vi "OAT Timebase Plot (Vector Data).vi"(0 "magnitudes":T3(array[cluster]) {"magnitude" format="%.2f"; "time/rev/rpm" format="%.2f"}, 2 "order to display":dbl=1.0 format="%.2f", 5 "phases [phase lag]":cluster{"time/rev/rpm":dbl[], "phase":dbl[]}[](array[cluster]) {"phase" format="%.2f"; "time/rev/rpm" format="%.2f"}, 7 "samples/rev wanted":i32=64, 9 "revolutions to display [rev]":cluster{"start":dbl, "duration":dbl}={"start"=0.0, "duration"=8.0} {"duration" format="%.2f"; "start" format="%.2f"}, 11 "error in (no error)":errorcluster, 13 "view":T2={"dB on? (F)"=FALSE, "unwrap phase? (T)"=TRUE, "unit in degree? (T)"=TRUE}, 14 "trigger pulse direction":u16(ring)=1 items=["positive going", "negative going"]) -> (4 "X axis":T1, 6 "Y axis":T1, 15 "error out":errorcluster)   [LabVIEW 2017]
doc: "Draws a timebase plot on an XY graph. You can use this polymorphic VI with unfiltered or filtered data. The unfiltered data comes from the <B>even angle signals</B> input, the filtered data from the <B>magnitudes</B> and <B>phases [phase lag]</B> inputs. The timebase plot displays the amplitude of a signal as a function of time and marks the tachometer trigger point on the plot. The data type you wire to the <B>even angle signals</B> input determines the polymorphic instance to use."
uses:
  <vilib>/addons/Sound and Vibration/Order Analysis/Backward Compatibility/SubVIs/oa_Timebase Plot Control.ctl
  <vilib>/addons/Sound and Vibration/Order Analysis/Resample Order Tracking/SoundVib_Resampling.lvlib
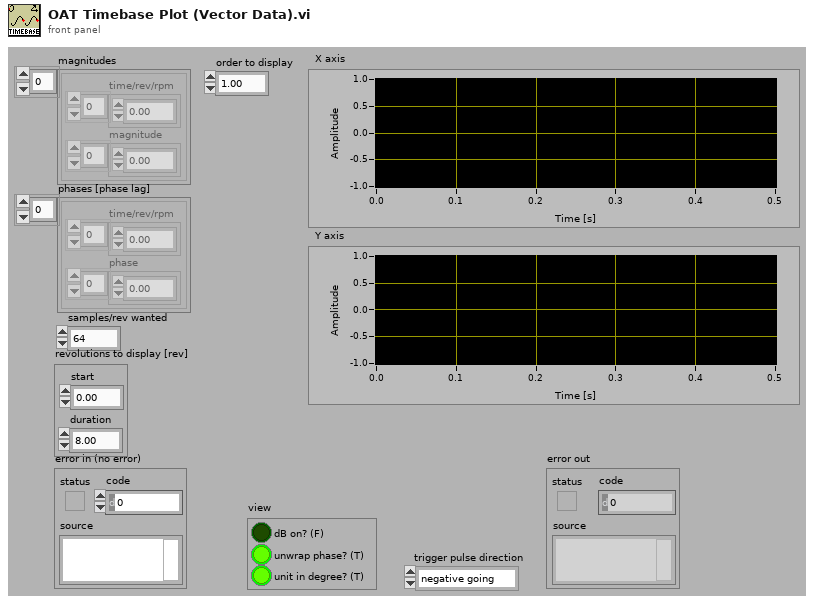
[diagram p1: front panel]
types:
  T1 = typedef "oa_Timebase Plot Control.ctl" = cluster{"X":dbl[], "Y":dbl[]}[]
  T2 = cluster{"dB on? (F)":bool, "unwrap phase? (T)":bool, "unit in degree? (T)":bool}
  T3 = cluster{"time/rev/rpm":dbl[], "magnitude":dbl[]}[]
  T4 = cluster{"interpolated pulse positions[s]":dbl[], "order waveform":dbl[]}
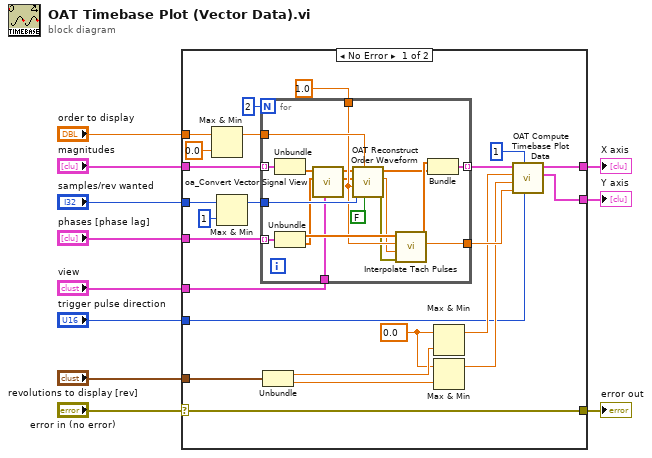
[diagram p0: block diagram]
diagram:
  n1 = case shown="No Error" "error in (no error)" {
    selector: "error in (no error)" -> [w24 w55]
    tunnel: [w24 w55] -> w10
    tunnel: [w20 w54] -> w4
    tunnel: [w19 w54] -> w5
    tunnel: "magnitudes" -> [w34 _]
    tunnel: "phases [phase lag]" -> [w33 _]
    tunnel: "order to display" -> [w32 _]
    tunnel: "samples/rev wanted" -> [w22 _]
    tunnel: "revolutions to display [rev]" -> [w18 _]
    tunnel: "trigger pulse direction" -> [w17 _]
    tunnel: "view" -> [w15 _]
    frame No Error {
      w25 = 0.0 ("y")
      n2 = Max & Min(x=w32, y=0.0 ("t")) -> (max(x,y)=w13:dbl)  [unwired: 1 out]
      n3 = Max & Min(x=w22, y=1 ("x")) -> (max(x,y)=w23:i32)  [unwired: 1 out]
      n4 = for {
        N: 2 -> [_]
        tunnel: w13 -> [w53]
        tunnel: 1.0 ("t") -> [w48]
        tunnel: w34 -> [w52] mode=indexing
        tunnel: w33 -> [w51] mode=indexing
        tunnel: w23 -> [w50]
        tunnel: [w45] -> w30
        tunnel: [w42] -> w14 mode=indexing
        tunnel: w15 -> [w37]
        n5 = Unbundle(w52) -> ("magnitude"=w41:dbl[])  [unwired: 1 out]
        n6 = Unbundle(w51) -> ("time/rev/rpm"=w49:dbl[], "phase"=w40:dbl[])
        n7 = call <vilib>:"oa_Convert Vector Signal View.vi"("view"=w37, "phase"=w40, "magnitude"=w41) -> ("phase out"=w38:dbl[], "magnitude out"=w39:dbl[])  [unwired: 7 in]
        n8 = call <vilib>:"OAT Reconstruct Order Waveform.vi"("unit in degree? (F)"=FALSE, "order"=w53, "samples/revolution wanted"=w50, "samples/revolution"=w48, "phase lag"=w38, "magnitude"=w39) -> ("error out"=w46:errorcluster, "actual samples/rev"=w47:dbl, "order waveform"=w43:dbl[])  [unwired: 3 in]
        n9 = call <vilib>:"Interpolate Tach Pulses.vi"("error in (no error)"=w46, "pulse/revolution wanted"=w47, "pulse/revolution (1)"=w48, "pulse positions [s]"=w49) -> ("new pulse/revolution"=w45:dbl, "interpolated pulse positions[s]"=w44:dbl[])  [unwired: 5 in, 1 out]
        n10 = Bundle("interpolated pulse positions[s]"=w44, "order waveform"=w43) -> (w42:T4)  [unwired: 1 in]
      }
      n11 = Unbundle(w18) -> ("start"=w26:dbl, "duration"=w27:dbl)
      n12 = Max & Min(x=w25, y=w26) -> (max(x,y)=w29:dbl)  [unwired: 1 out]
      n13 = Max & Min(x=w25, y=w27) -> (max(x,y)=w28:dbl)  [unwired: 1 out]
      n14 = call <vilib>:"OAT Compute Timebase Plot Data.vi"("trigger pulse direction"=w17, "tach duty"=1, "actual samples/rev"=w30, "revolutions"=w28, "start"=w29, "timebase plot in"=w14) -> ("Y axis out"=w19:cluster{dbl[], dbl[]}[], "X axis out"=w20:cluster{dbl[], dbl[]}[])  [unwired: 4 in]
    }
    frame Error {
      w54 = cluster{"X":dbl[], "Y":dbl[]}[] [] ("X axis Plot")
    }
  }
  "error out" <- w10
  "Y axis" <- w5
  "X axis" <- w4
